vi "Get Short Help.vi"(8 "error in (no error)":errorcluster, 11 "Action in":refnum<class "Action.lvclass">) -> (0 "error out":errorcluster, 2 "Short Help":string, 3 "Action out":refnum<class "Action.lvclass">)   [LabVIEW 2020, in "neg-pkg.lvlib" / "Action.lvclass"]
uses:
  Action.lvclass
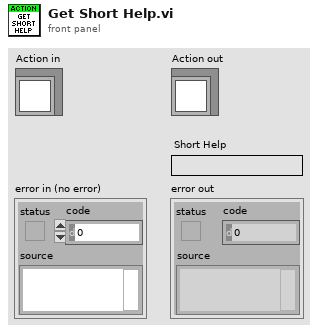
[diagram p1: front panel]
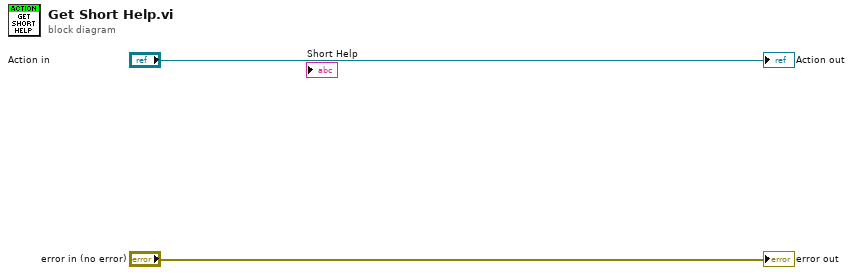
[diagram p0: block diagram]
diagram:
  "error out" <- "error in (no error)"
  "Action out" <- "Action in"
